vi "release queues.vi"(7 "power monitor queue out":refnum<queue>, 8 "error in (no error)":errorcluster, 9 "register monitor queue out":refnum<queue>, 10 "i2c queue out":refnum<queue>, 11 "image queue out":refnum<queue>) -> (0 "error out":errorcluster)   [LabVIEW 2025, in "Automotive Vision.lvclass"]
uses:
  Automotive Vision.lvclass
  Automotive Vision.lvclass/Automotive Vision.ctl
  regitster_value.ctl
  power.ctl
  image.ctl
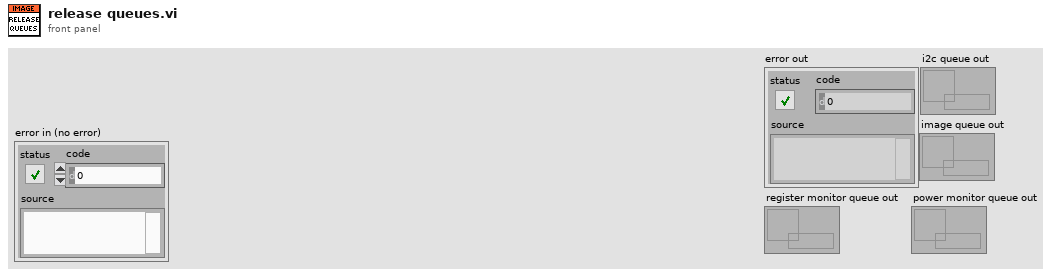
[diagram p1: front panel]
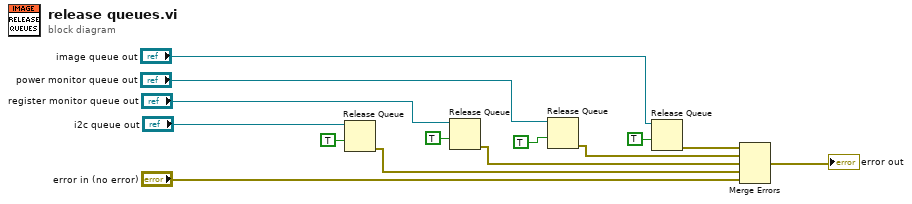
[diagram p0: block diagram]
diagram:
  n1 = Release Queue(queue="i2c queue out", force destroy? (F)=TRUE) -> (error out=w4:errorcluster)  [unwired: 1 in, 2 out]
  n2 = Release Queue(queue="register monitor queue out", force destroy? (F)=TRUE) -> (error out=w3:errorcluster)  [unwired: 1 in, 2 out]
  n3 = Release Queue(queue="power monitor queue out", force destroy? (F)=TRUE) -> (error out=w2:errorcluster)  [unwired: 1 in, 2 out]
  n4 = Release Queue(queue="image queue out", force destroy? (F)=TRUE) -> (error out=w1:errorcluster)  [unwired: 1 in, 2 out]
  n5 = Merge Errors(w1, w2, w3, w4, "error in (no error)") -> (→"error out":errorcluster)
